vi "Header data_Cnsl.vi"(0 "base path":path=path "C:/", 5 "prompt (Create Folder)":string="logsConsole", 7 "file name":string, 11 "Error In":errorcluster) -> (4 "refnum out":refnum<file>, 15 "error out":errorcluster)   [LabVIEW 2018]
uses:
  Global_1259.vi
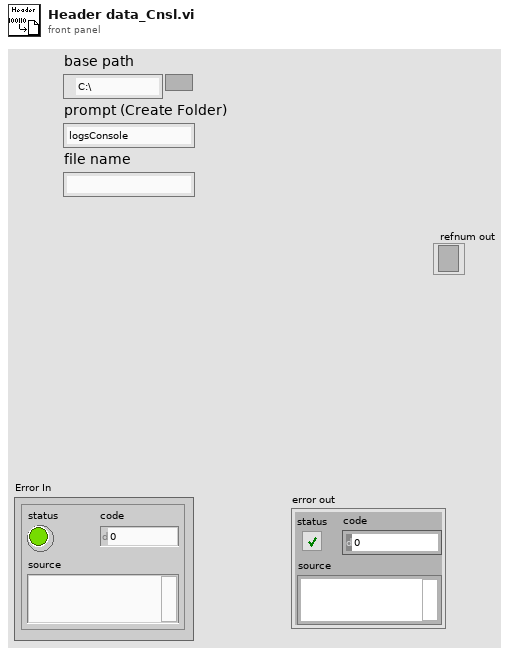
[diagram p1: front panel]
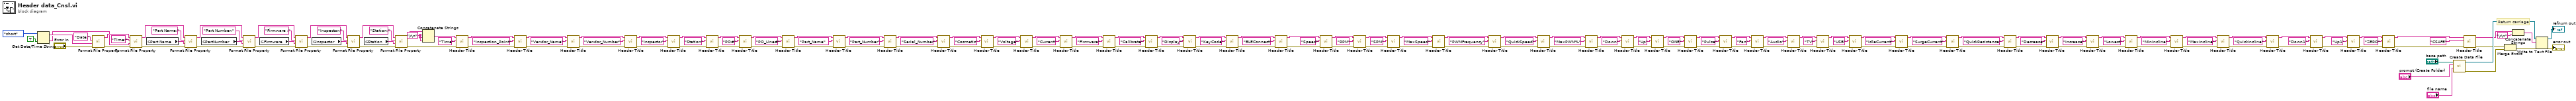
[diagram p0: block diagram]
diagram:
  w43 = "\r\n"
  # "Return carriage"
  n1 = Get Date/Time String(date format (0)=enum16{"short", "long", "abbreviated"}."short", want seconds? (F)=TRUE) -> (date string=w54:string, time string=w53:string)  [unwired: 1 in]
  n2 = call "Format File Property.vi"("Error In"="Error In", "File Property Value"=w54, "File Property Name"="Date:") -> ("Error Out"=w183:errorcluster, "String out"=w127:string)  [unwired: 7 in]
  n3 = call "Format File Property.vi"("Error In"=w183, "File Property Value"=w53, "File Property Name"="Time:", "String in"=w127) -> ("Error Out"=w46:errorcluster, "String out"=w47:string)  [unwired: 6 in]
  n4 = global read "Global_1259.vi" "Part Name"() -> (w115:string)
  n5 = call "Format File Property.vi"("Error In"=w46, "File Property Value"=w115, "File Property Name"="Part Name:", "String in"=w47) -> ("Error Out"=w178:errorcluster, "String out"=w125:string)  [unwired: 6 in]
  n6 = global read "Global_1259.vi" "PartNumber"() -> (w114:string)
  n7 = call "Format File Property.vi"("Error In"=w178, "File Property Value"=w114, "File Property Name"="Part Number:", "String in"=w125) -> ("Error Out"=w184:errorcluster, "String out"=w124:string)  [unwired: 6 in]
  n8 = global read "Global_1259.vi" "Firmware"() -> (w113:string)
  n9 = call "Format File Property.vi"("Error In"=w184, "File Property Value"=w113, "File Property Name"="Firmware :", "String in"=w124) -> ("Error Out"=w41:errorcluster, "String out"=w42:string)  [unwired: 6 in]
  n10 = global read "Global_1259.vi" "Inspector"() -> (w39:string)
  n11 = call "Format File Property.vi"("Error In"=w41, "File Property Value"=w39, "File Property Name"="Inspector:", "String in"=w42) -> ("Error Out"=w182:errorcluster, "String out"=w126:string)  [unwired: 6 in]
  n12 = global read "Global_1259.vi" "Station"() -> (w38:string)
  n13 = call "Format File Property.vi"("Error In"=w182, "File Property Value"=w38, "File Property Name"="Station:", "String in"=w126) -> ("Error Out"=w11:errorcluster, "String out"=w40:string)  [unwired: 6 in]
  n14 = Concatenate Strings(w40, w43, w43, w43) -> (w12:string)
  n15 = call "Header Title.vi"("Error In"=w11, "Header Title"="Time", "String in"=w12) -> ("Error Out"=w8:errorcluster, "String out"=w7:string)  [unwired: 7 in]
  n16 = call "Header Title.vi"("Error In"=w8, "Header Title"="Inspection_Point", "String in"=w7) -> ("Error Out"=w9:errorcluster, "String out"=w10:string)  [unwired: 7 in]
  n17 = call "Header Title.vi"("Error In"=w9, "Header Title"="Vendor_Name" ("File Property Name"), "String in"=w10) -> ("Error Out"=w28:errorcluster, "String out"=w36:string)  [unwired: 7 in]
  n18 = call "Header Title.vi"("Error In"=w28, "Header Title"="Vendor_Number" ("File Property Name"), "String in"=w36) -> ("Error Out"=w27:errorcluster, "String out"=w29:string)  [unwired: 7 in]
  n19 = call "Header Title.vi"("Error In"=w27, "Header Title"="Inspector" ("File Property Name"), "String in"=w29) -> ("Error Out"=w26:errorcluster, "String out"=w32:string)  [unwired: 7 in]
  n20 = call "Header Title.vi"("Error In"=w26, "Header Title"="Station" ("File Property Name"), "String in"=w32) -> ("Error Out"=w25:errorcluster, "String out"=w31:string)  [unwired: 7 in]
  n21 = call "Header Title.vi"("Error In"=w25, "Header Title"="PO#" ("File Property Name"), "String in"=w31) -> ("Error Out"=w19:errorcluster, "String out"=w18:string)  [unwired: 7 in]
  n22 = call "Header Title.vi"("Error In"=w19, "Header Title"="PO_Line#", "String in"=w18) -> ("Error Out"=w16:errorcluster, "String out"=w17:string)  [unwired: 7 in]
  n23 = call "Header Title.vi"("Error In"=w16, "Header Title"="Part_Name" ("File Property Name"), "String in"=w17) -> ("Error Out"=w21:errorcluster, "String out"=w23:string)  [unwired: 7 in]
  n24 = call "Header Title.vi"("Error In"=w21, "Header Title"="Part_Number" ("File Property Name"), "String in"=w23) -> ("Error Out"=w14:errorcluster, "String out"=w13:string)  [unwired: 7 in]
  n25 = call "Header Title.vi"("Error In"=w14, "Header Title"="Serial_Number" ("string"), "String in"=w13) -> ("Error Out"=w131:errorcluster, "String out"=w130:string)  [unwired: 7 in]
  n26 = call "Header Title.vi"("Error In"=w131, "Header Title"="Cosmetic", "String in"=w130) -> ("Error Out"=w135:errorcluster, "String out"=w134:string)  [unwired: 7 in]
  n27 = call "Header Title.vi"("Error In"=w135, "Header Title"="Voltage", "String in"=w134) -> ("Error Out"=w128:errorcluster, "String out"=w129:string)  [unwired: 7 in]
  n28 = call "Header Title.vi"("Error In"=w128, "Header Title"="Current" ("string"), "String in"=w129) -> ("Error Out"=w97:errorcluster, "String out"=w98:string)  [unwired: 7 in]
  n29 = call "Header Title.vi"("Error In"=w97, "Header Title"="Firmware" ("string"), "String in"=w98) -> ("Error Out"=w96:errorcluster, "String out"=w95:string)  [unwired: 7 in]
  n30 = call "Header Title.vi"("Error In"=w96, "Header Title"="Calibrate" ("string"), "String in"=w95) -> ("Error Out"=w140:errorcluster, "String out"=w161:string)  [unwired: 7 in]
  n31 = call "Header Title.vi"("Error In"=w140, "Header Title"="Display" ("string"), "String in"=w161) -> ("Error Out"=w72:errorcluster, "String out"=w71:string)  [unwired: 7 in]
  n32 = call "Header Title.vi"("Error In"=w72, "Header Title"="KeyCode", "String in"=w71) -> ("Error Out"=w73:errorcluster, "String out"=w70:string)  [unwired: 7 in]
  n33 = call "Header Title.vi"("Error In"=w73, "Header Title"="BLEConnect", "String in"=w70) -> ("Error Out"=w60:errorcluster, "String out"=w59:string)  [unwired: 7 in]
  n34 = call "Header Title.vi"("Error In"=w60, "Header Title"="Speed", "String in"=w59) -> ("Error Out"=w58:errorcluster, "String out"=w57:string)  [unwired: 7 in]
  n35 = call "Header Title.vi"("Error In"=w58, "Header Title"="RPM", "String in"=w57) -> ("Error Out"=w3:errorcluster, "String out"=w4:string)  [unwired: 7 in]
  n36 = call "Header Title.vi"("Error In"=w3, "Header Title"="SPM", "String in"=w4) -> ("Error Out"=w1:errorcluster, "String out"=w2:string)  [unwired: 7 in]
  n37 = call "Header Title.vi"("Error In"=w1, "Header Title"="MaxSpeed", "String in"=w2) -> ("Error Out"=w153:errorcluster, "String out"=w156:string)  [unwired: 7 in]
  n38 = call "Header Title.vi"("Error In"=w153, "Header Title"="PWMFrequency", "String in"=w156) -> ("Error Out"=w117:errorcluster, "String out"=w118:string)  [unwired: 7 in]
  n39 = call "Header Title.vi"("Error In"=w117, "Header Title"="QuickSpeed", "String in"=w118) -> ("Error Out"=w87:errorcluster, "String out"=w88:string)  [unwired: 7 in]
  n40 = call "Header Title.vi"("Error In"=w87, "Header Title"="MaxPWM%" ("Measured Data"), "String in"=w88) -> ("Error Out"=w139:errorcluster, "String out"=w160:string)  [unwired: 7 in]
  n41 = call "Header Title.vi"("Error In"=w139, "Header Title"="Down" ("Measured Data"), "String in"=w160) -> ("Error Out"=w136:errorcluster, "String out"=w137:string)  [unwired: 7 in]
  n42 = call "Header Title.vi"("Error In"=w136, "Header Title"="Up", "String in"=w137) -> ("Error Out"=w154:errorcluster, "String out"=w157:string)  [unwired: 7 in]
  n43 = call "Header Title.vi"("Error In"=w154, "Header Title"="ONE", "String in"=w157) -> ("Error Out"=w85:errorcluster, "String out"=w86:string)  [unwired: 7 in]
  n44 = call "Header Title.vi"("Error In"=w85, "Header Title"="Pulse", "String in"=w86) -> ("Error Out"=w152:errorcluster, "String out"=w155:string)  [unwired: 7 in]
  n45 = call "Header Title.vi"("Error In"=w152, "Header Title"="Fan", "String in"=w155) -> ("Error Out"=w119:errorcluster, "String out"=w120:string)  [unwired: 7 in]
  n46 = call "Header Title.vi"("Error In"=w119, "Header Title"="Audio", "String in"=w120) -> ("Error Out"=w122:errorcluster, "String out"=w123:string)  [unwired: 7 in]
  n47 = call "Header Title.vi"("Error In"=w122, "Header Title"="TV", "String in"=w123) -> ("Error Out"=w144:errorcluster, "String out"=w145:string)  [unwired: 7 in]
  n48 = call "Header Title.vi"("Error In"=w144, "Header Title"="USB", "String in"=w145) -> ("Error Out"=w92:errorcluster, "String out"=w91:string)  [unwired: 7 in]
  n49 = call "Header Title.vi"("Error In"=w92, "Header Title"="IdleCurrent" ("Measured Data"), "String in"=w91) -> ("Error Out"=w64:errorcluster, "String out"=w65:string)  [unwired: 7 in]
  n50 = call "Header Title.vi"("Error In"=w64, "Header Title"="SurgeCurrent", "String in"=w65) -> ("Error Out"=w63:errorcluster, "String out"=w62:string)  [unwired: 7 in]
  n51 = call "Header Title.vi"("Error In"=w63, "Header Title"="QuickResistance", "String in"=w62) -> ("Error Out"=w102:errorcluster, "String out"=w103:string)  [unwired: 7 in]
  n52 = call "Header Title.vi"("Error In"=w102, "Header Title"="Decrease", "String in"=w103) -> ("Error Out"=w89:errorcluster, "String out"=w90:string)  [unwired: 7 in]
  n53 = call "Header Title.vi"("Error In"=w89, "Header Title"="Increase" ("Measured Data"), "String in"=w90) -> ("Error Out"=w66:errorcluster, "String out"=w67:string)  [unwired: 7 in]
  n54 = call "Header Title.vi"("Error In"=w66, "Header Title"="Lowest", "String in"=w67) -> ("Error Out"=w49:errorcluster, "String out"=w50:string)  [unwired: 7 in]
  n55 = call "Header Title.vi"("Error In"=w49, "Header Title"="MinIncline", "String in"=w50) -> ("Error Out"=w52:errorcluster, "String out"=w51:string)  [unwired: 7 in]
  n56 = call "Header Title.vi"("Error In"=w52, "Header Title"="MaxIncline", "String in"=w51) -> ("Error Out"=w76:errorcluster, "String out"=w77:string)  [unwired: 7 in]
  n57 = call "Header Title.vi"("Error In"=w76, "Header Title"="QuickIncline" ("Measured Data"), "String in"=w77) -> ("Error Out"=w84:errorcluster, "String out"=w83:string)  [unwired: 7 in]
  n58 = call "Header Title.vi"("Error In"=w84, "Header Title"="Down1", "String in"=w83) -> ("Error Out"=w80:errorcluster, "String out"=w79:string)  [unwired: 7 in]
  n59 = call "Header Title.vi"("Error In"=w80, "Header Title"="Up1", "String in"=w79) -> ("Error Out"=w74:errorcluster, "String out"=w75:string)  [unwired: 7 in]
  n60 = call "Header Title.vi"("Error In"=w74, "Header Title"="ZERO", "String in"=w75) -> ("Error Out"=w93:errorcluster, "String out"=w94:string)  [unwired: 7 in]
  n61 = call "Create Data File.vi"("file name"="file name", "prompt (Create Folder)"="prompt (Create Folder)", "base path"="base path") -> ("Error Out"=w179:errorcluster, "File Refnum"=w181:refnum<file>)  [unwired: 7 in]
  n62 = call "Header Title.vi"("Error In"=w93, "Header Title"="CSAFE", "String in"=w94) -> ("Error Out"=w112:errorcluster, "String out"=w111:string)  [unwired: 7 in]
  n63 = Merge Errors(w112, w179) -> (w180:errorcluster)
  n64 = Concatenate Strings(w111, "\r\n") -> (w158:string)
  n65 = Write to Text File(file (use dialog)=w181, text=w158, error in=w180) -> (refnum out=→"refnum out":refnum<file>, error out=→"error out":errorcluster)  [unwired: 1 in, 1 out]
